vi "AOL Properties parser.vi"(0 "AOL Properties":T4={"AOD 1 thickness (mm)"=118.0, "AOD 2 thickness (mm)"=115.0, "AOD 3 thickness (mm)"=110.0, "AOD 4 thickness (mm)"=135.0, "AOD 5 thickness (mm)"=135.0, "AOD 6 thickness (mm)"=135.0, "AOD 1-2 separation (mm)"=15.0, "AOD 2-3 separation (mm)"=15.0, "AOD 3-4 separation (mm)"=15.0, "AOD 4-5 separation (mm)"=15.0, "AOD 5-6 separation (mm)"=15.0, "AOD 1 X Offset"=15.0, "AOD 2 X Offset"=1.0, "AOD 3 X Offset"=1.0, "AOD 4 X Offset"=1.0, "AOD 1 Y Offset"=1.0, "AOD 2 Y Offset"=1.0, "AOD 3 Y Offset"=1.0, "AOD 4 Y Offset"=1.0, "AOD 1 X Direction"=0.0, "AOD 2 X Direction"=0.0, "AOD 3 X Direction"=0.0, "AOD 4 X Direction"=0.0, "AOD 1 Y Direction"=1.0, "AOD 2 Y Direction"=0.0, "AOD 3 Y Direction"=0.0023, "AOD 4 Y Direction"=0.0046, "AOD 1 Centre (mm)"=15.0, "AOD 2 Centre (mm)"=50.0, "AOD 3 Centre (mm)"=50.0, "AOD 4 Centre (mm)"=50.0, "Timing Offset AOD 1"=0.0, "Timing Offset AOD 2"=0.0, "Timing Offset AOD 3"=0.0, "Timing Offset AOD 4"=0.0, "AOD Optical offset 1"=20000.0, "AOD Optical offset 2"=20000.0, "AOL aperture (mm)"=15.0, "AOL centre wavelength (nm)"=1.0, "AOL centre frequency (MHz)"=1.0, "Diffraction mode"=1.0, "Crystal length (mm)"=0.0, "Acoustic velocity (m/s)"=1.0, "Pair deflection ratio"=1.0, "AOD fill time (us)"=1.0, "AOD Ord. Refractive index"=2.22, "AOD ExtraOrd. Refractive index"=2.22}) -> (14 "Keys setup.DBL":T2=[{"key"="Control FPGA.Clock Freq (MHz)", "Save?"=TRUE, "Default"=240.0}, {"key"="DAQ FPGA.Clock Freq (MHz)", "Save?"=TRUE, "Default"=240.0}], 15 "Values.DBL":dbl[](array[numeric]), 16 "Keys setup.String":T3=[{"key"="Control FPGA.MAC address", "Save?"=TRUE, "Default"="AABBCCDDEEFF"}, {"key"="DAQ FPGA.Target", "Save?"=TRUE, "Default"="RIO0"}, {"key"="XY Stage.COM port", "Save?"=TRUE, "Default"="COM7"}, {"key"="DAQmx Chan.Pockels Control", "Save?"=TRUE, "Default"=""}, {"key"="DAQmx Chan.Hard Shutter", "Save?"=TRUE, "Default"=""}, {"key"="DAQmx Chan.PMT 1", "Save?"=TRUE, "Default"=""}, {"key"="DAQmx Chan.PMT 2", "Save?"=TRUE, "Default"=""}, {"key"="DAQmx Chan.Encoder Trigger", "Save?"=TRUE, "Default"=""}, {"key"="DAQmx Chan.Optional Trigger 1", "Save?"=TRUE, "Default"=""}, {"key"="DAQmx Chan.Optional Trigger 2", "Save?"=TRUE, "Default"=""}, {"key"="DAQmx Chan.Optional Trigger 3", "Save?"=TRUE, "Default"=""}], 17 "Values.Strings":string[](array[string]), 18 "Keys setup.Boolean":T1, 19 "Values.Boolean":bool[](array[boolean]))   [LabVIEW 2017]
uses:
  Typedefs/AOL Properties Cluster.ctl
  Typedefs/Ini file interface (String).ctl
  Typedefs/Ini file interface (DBL).ctl
  Typedefs/Ini file interface (Boolean).ctl
panel:
  # "NOTES:\n1. \"Control FPGA.Ethernet port\" is detected automatically. It is not saved/loaded from file.\n2. \"Control FPGA.Ethernet Opened\" is detected automatically. It is not saved/loaded from file."
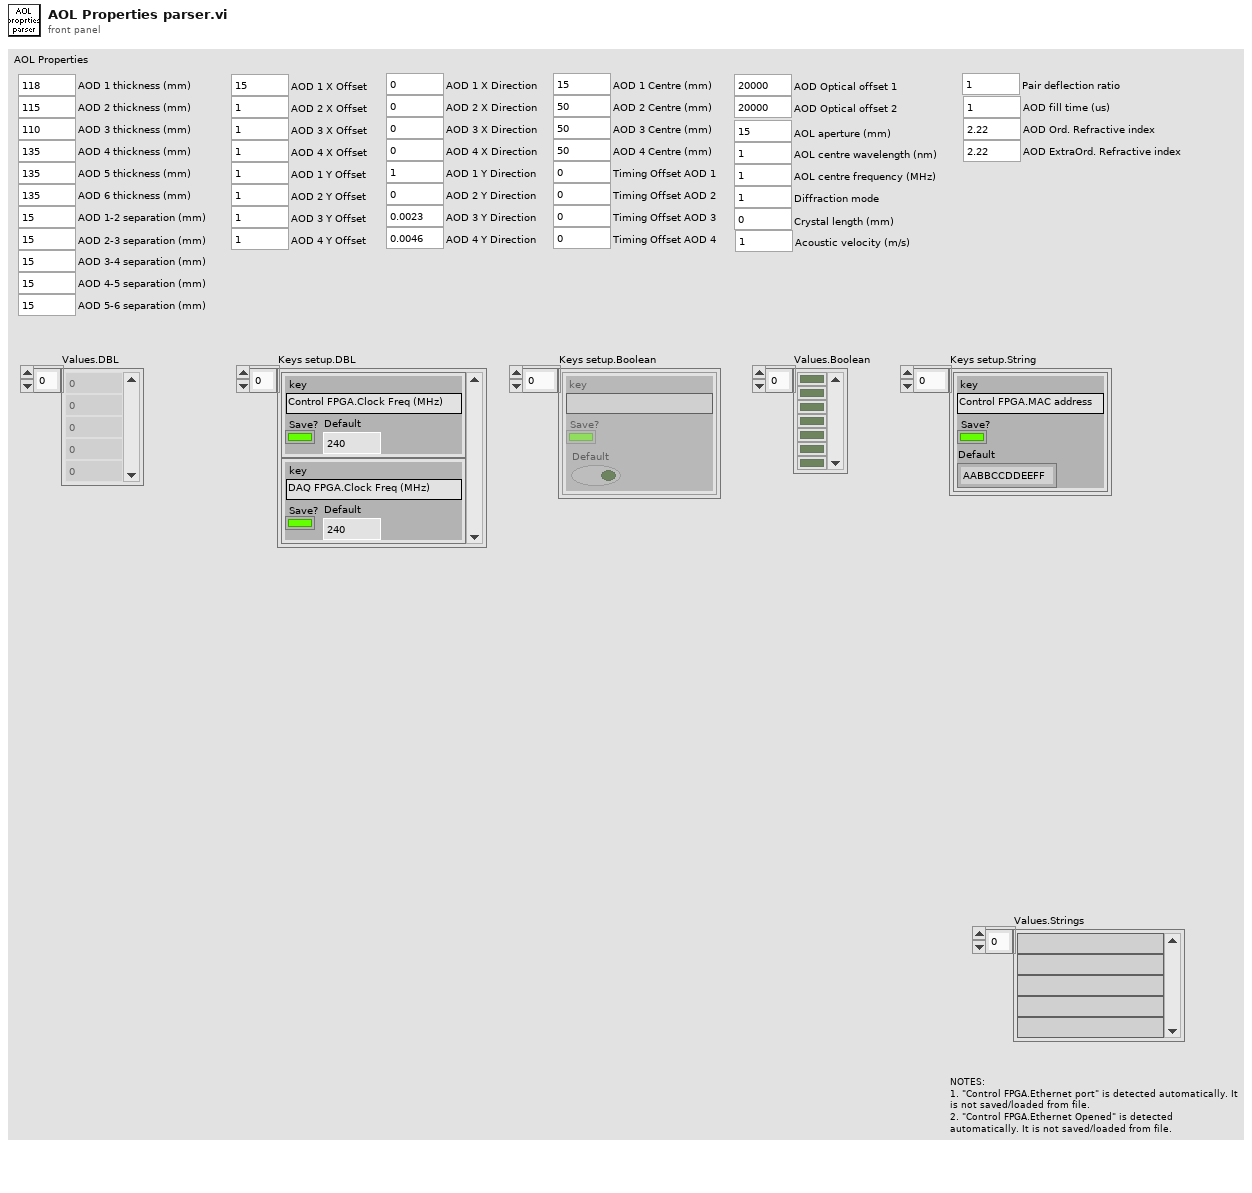
[diagram p1: front panel]
types:
  T1 = typedef "Ini file interface (Boolean).ctl" = cluster{"key":string, "Save?":bool, "Default":bool}[]
  T2 = typedef "Ini file interface (DBL).ctl" = cluster{"key":string, "Save?":bool, "Default":dbl}[]
  T3 = typedef "Ini file interface (String).ctl" = cluster{"key":string, "Save?":bool, "Default":string}[]
  T4 = typedef "AOL Properties Cluster.ctl" = cluster{"AOD 1 thickness (mm)":dbl, "AOD 2 thickness (mm)":dbl, "AOD 3 thickness (mm)":dbl, "AOD 4 thickness (mm)":dbl, "AOD 5 thickness (mm)":dbl, "AOD 6 thickness (mm)":dbl, "AOD 1-2 separation (mm)":dbl, "AOD 2-3 separation (mm)":dbl, "AOD 3-4 separation (mm)":dbl, "AOD 4-5 separation (mm)":dbl, "AOD 5-6 separation (mm)":dbl, "AOD 1 X Offset":dbl, "AOD 2 X Offset":dbl, "AOD 3 X Offset":dbl, "AOD 4 X Offset":dbl, "AOD 1 Y Offset":dbl, "AOD 2 Y Offset":dbl, "AOD 3 Y Offset":dbl, "AOD 4 Y Offset":dbl, "AOD 1 X Direction":dbl, "AOD 2 X Direction":dbl, "AOD 3 X Direction":dbl, "AOD 4 X Direction":dbl, "AOD 1 Y Direction":dbl, "AOD 2 Y Direction":dbl, "AOD 3 Y Direction":dbl, "AOD 4 Y Direction":dbl, "AOD 1 Centre (mm)":dbl, "AOD 2 Centre (mm)":dbl, "AOD 3 Centre (mm)":dbl, "AOD 4 Centre (mm)":dbl, "Timing Offset AOD 1":dbl, "Timing Offset AOD 2":dbl, "Timing Offset AOD 3":dbl, "Timing Offset AOD 4":dbl, "AOD Optical offset 1":dbl, "AOD Optical offset 2":dbl, "AOL aperture (mm)":dbl, "AOL centre wavelength (nm)":dbl, "AOL centre frequency (MHz)":dbl, "Diffraction mode":dbl, "Crystal length (mm)":dbl, "Acoustic velocity (m/s)":dbl, "Pair deflection ratio":dbl, "AOD fill time (us)":dbl, "AOD Ord. Refractive index":dbl, "AOD ExtraOrd. Refractive index":dbl}
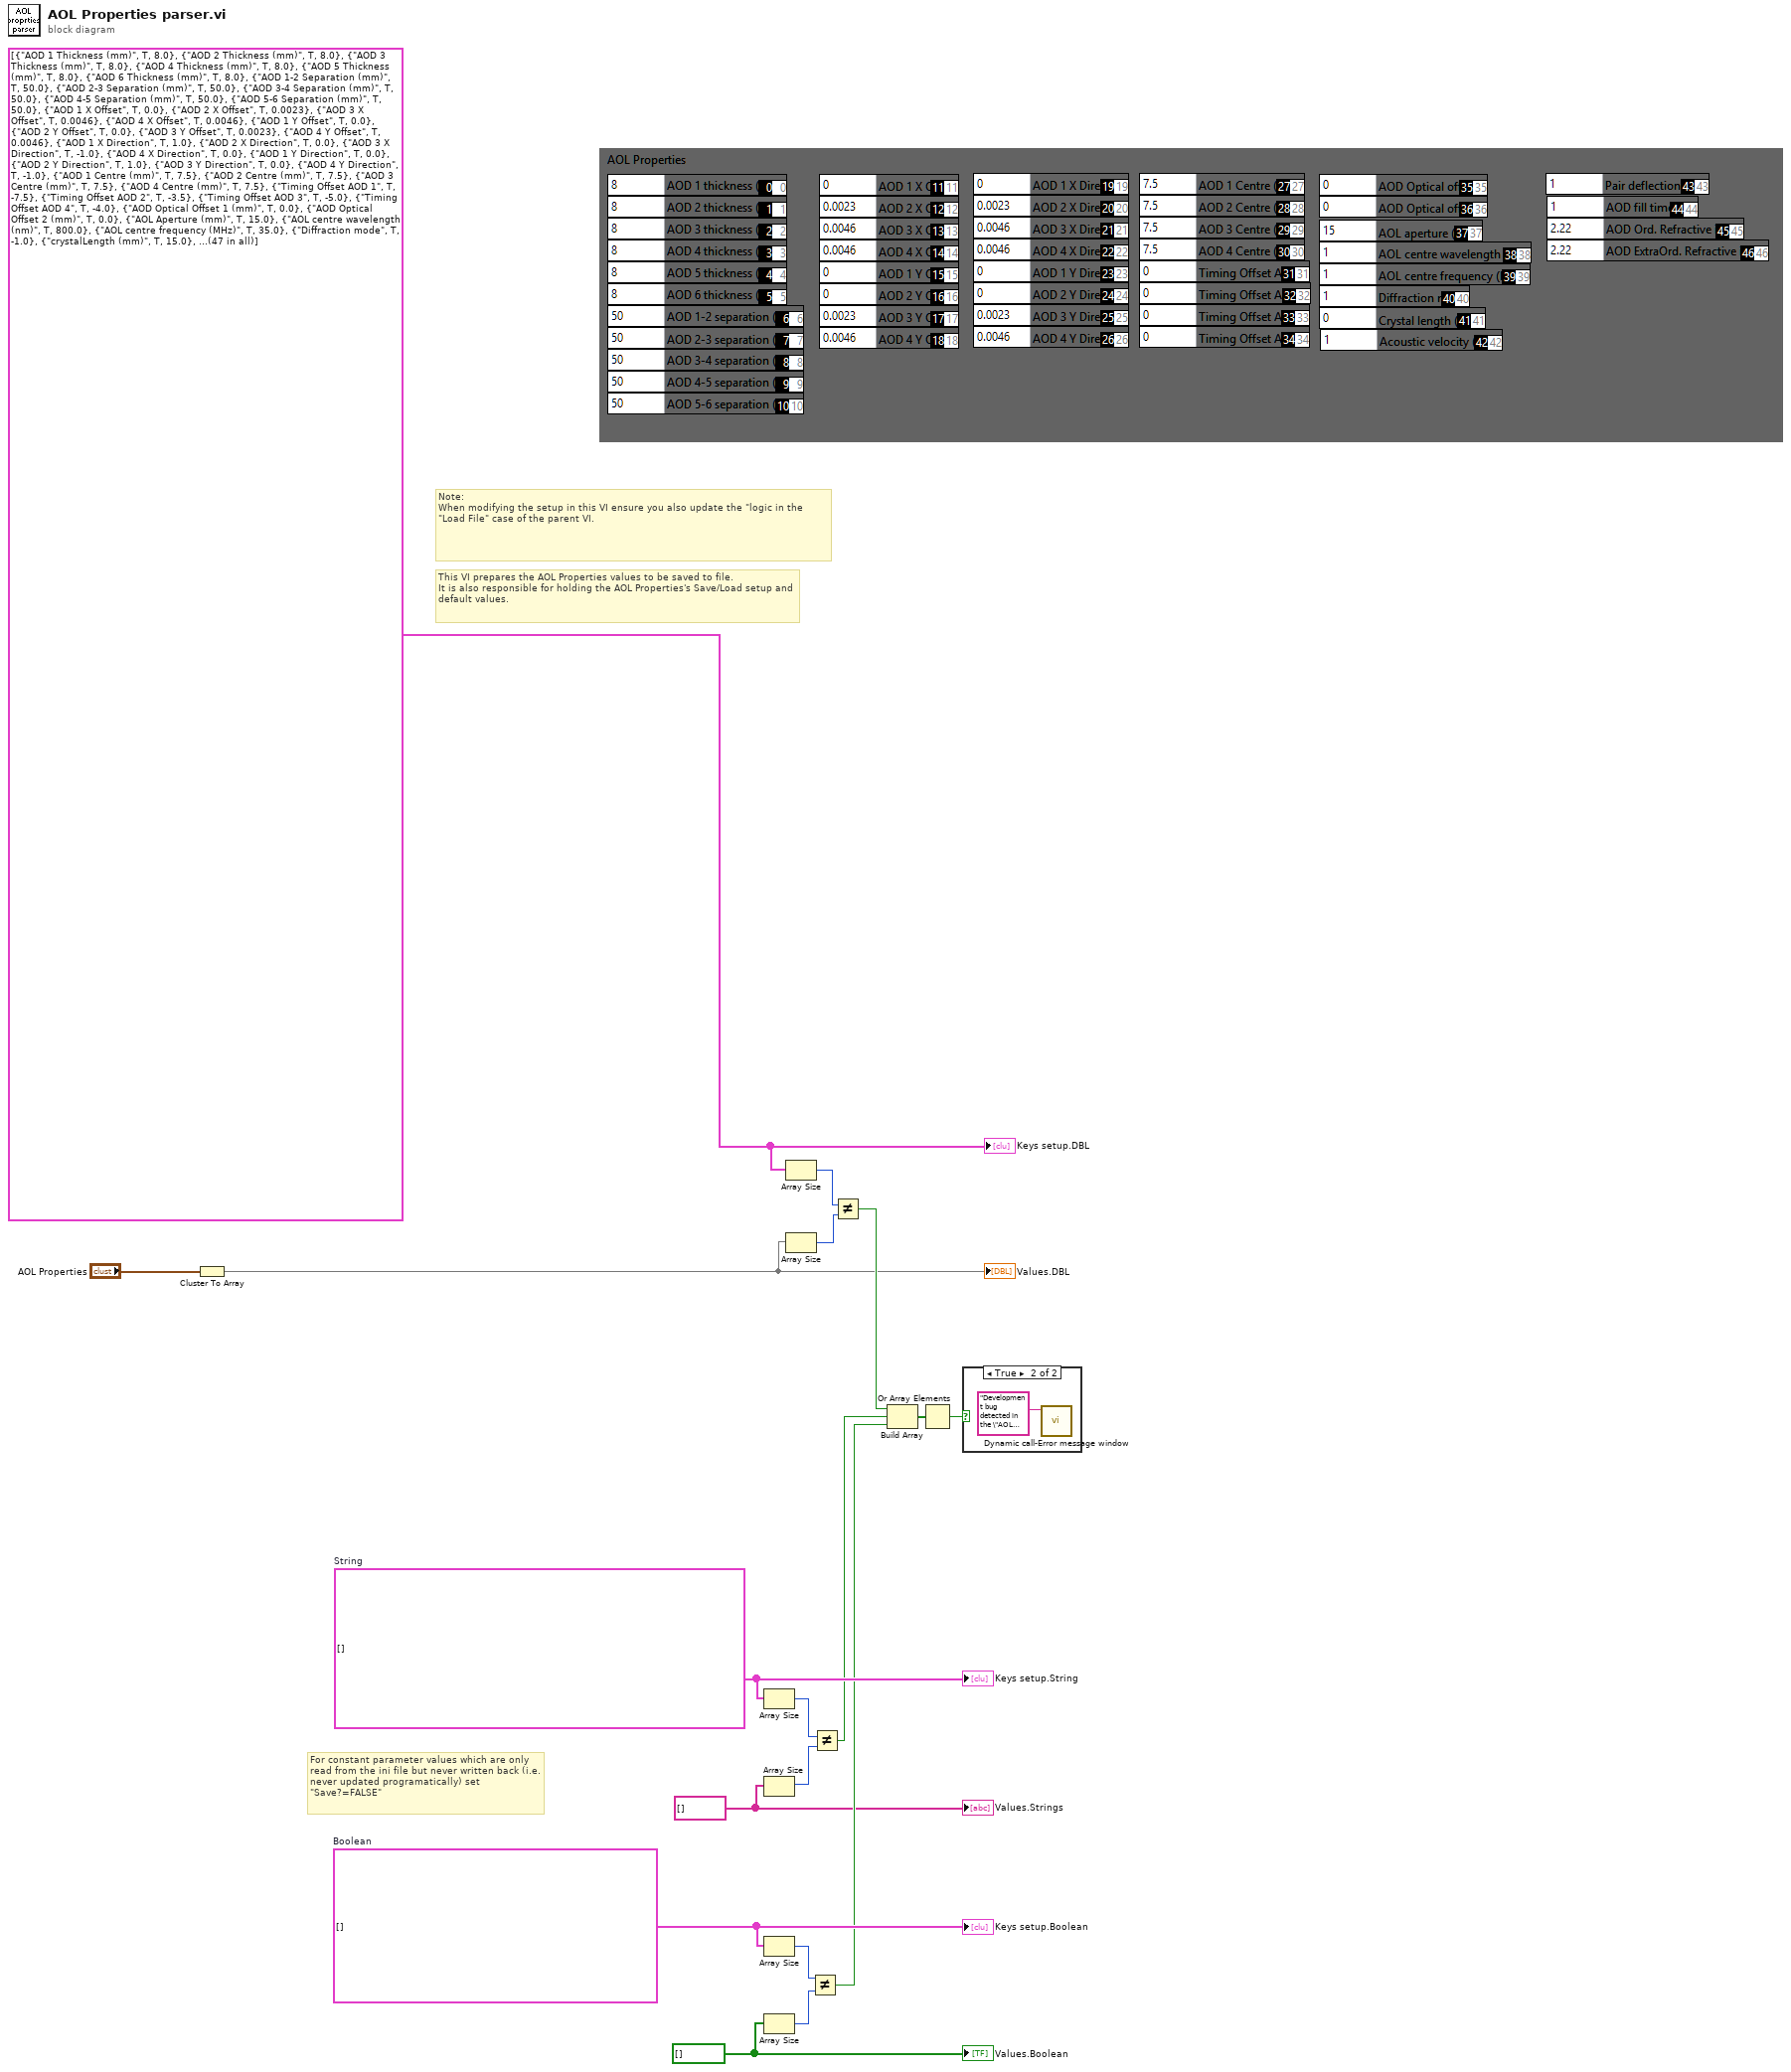
[diagram p0: block diagram]
diagram:
  w3 = T2 [{"key"="AOD 1 Thickness (mm)", "Save?"=TRUE, "Default"=8.0}, {"key"="AOD 2 Thickness (mm)", "Save?"=TRUE, "Default"=8.0}, {"key"="AOD 3 Thickness (mm)", "Save?"=TRUE, "Default"=8.0}, {"key"="AOD 4 Thickness (mm)", "Save?"=TRUE, "Default"=8.0}, {"key"="AOD 5 Thickness (mm)", "Save?"=TRUE, "Default"=8.0}, {"key"="AOD 6 Thickness (mm)", "Save?"=TRUE, "Default"=8.0}, {"key"="AOD 1-2 Separation (mm)", "Save?"=TRUE, "Default"=50.0}, {"key"="AOD 2-3 Separation (mm)", "Save?"=TRUE, "Default"=50.0}, {"key"="AOD 3-4 Separation (mm)", "Save?"=TRUE, "Default"=50.0}, {"key"="AOD 4-5 Separation (mm)", "Save?"=TRUE, "Default"=50.0}, {"key"="AOD 5-6 Separation (mm)", "Save?"=TRUE, "Default"=50.0}, {"key"="AOD 1 X Offset", "Save?"=TRUE, "Default"=0.0}, {"key"="AOD 2 X Offset", "Save?"=TRUE, "Default"=0.0023}, {"key"="AOD 3 X Offset", "Save?"=TRUE, "Default"=0.0046}, {"key"="AOD 4 X Offset", "Save?"=TRUE, "Default"=0.0046}, {"key"="AOD 1 Y Offset", "Save?"=TRUE, "Default"=0.0}, {"key"="AOD 2 Y Offset", "Save?"=TRUE, "Default"=0.0}, {"key"="AOD 3 Y Offset", "Save?"=TRUE, "Default"=0.0023}, {"key"="AOD 4 Y Offset", "Save?"=TRUE, "Default"=0.0046}, {"key"="AOD 1 X Direction", "Save?"=TRUE, "Default"=1.0}, {"key"="AOD 2 X Direction", "Save?"=TRUE, "Default"=0.0}, {"key"="AOD 3 X Direction", "Save?"=TRUE, "Default"=-1.0}, {"key"="AOD 4 X Direction", "Save?"=TRUE, "Default"=0.0}, {"key"="AOD 1 Y Direction", "Save?"=TRUE, "Default"=0.0}, {"key"="AOD 2 Y Direction", "Save?"=TRUE, "Default"=1.0}, {"key"="AOD 3 Y Direction", "Save?"=TRUE, "Default"=0.0}, {"key"="AOD 4 Y Direction", "Save?"=TRUE, "Default"=-1.0}, {"key"="AOD 1 Centre (mm)", "Save?"=TRUE, "Default"=7.5}, {"key"="AOD 2 Centre (mm)", "Save?"=TRUE, "Default"=7.5}, {"key"="AOD 3 Centre (mm)", "Save?"=TRUE, "Default"=7.5}, {"key"="AOD 4 Centre (mm)", "Save?"=TRUE, "Default"=7.5}, {"key"="Timing Offset AOD 1", "Save?"=TRUE, "Default"=-7.5}, {"key"="Timing Offset AOD 2", "Save?"=TRUE, "Default"=-3.5}, {"key"="Timing Offset AOD 3", "Save?"=TRUE, "Default"=-5.0}, {"key"="Timing Offset AOD 4", "Save?"=TRUE, "Default"=-4.0}, {"key"="AOD Optical Offset 1 (mm)", "Save?"=TRUE, "Default"=0.0}, {"key"="AOD Optical Offset 2 (mm)", "Save?"=TRUE, "Default"=0.0}, {"key"="AOL Aperture (mm)", "Save?"=TRUE, "Default"=15.0}, {"key"="AOL centre wavelength (nm)", "Save?"=TRUE, "Default"=800.0}, {"key"="AOL centre frequency (MHz)", "Save?"=TRUE, "Default"=35.0}, {"key"="Diffraction mode", "Save?"=TRUE, "Default"=-1.0}, {"key"="crystalLength (mm)", "Save?"=TRUE, "Default"=15.0}, {"key"="Acoustic velocity (m/s)", "Save?"=TRUE, "Default"=613.0}, {"key"="Pair Deflection Ratio", "Save?"=TRUE, "Default"=1.0}, {"key"="AOD fill time (us)", "Save?"=TRUE, "Default"=24.5}, {"key"="AOD Ord. Refractive index", "Save?"=TRUE, "Default"=2.22}, {"key"="AOD ExtraOrd. Refractive index", "Save?"=TRUE, "Default"=2.44}] ("DBL 3")
  w4 = bool[] [] ("appended array")
  w5 = string[] [] ("appended array")
  w17 = T1 []  # Boolean
  w18 = T3 []  # String
  # "Note:\nWhen modifying the setup in this VI ensure you also update the \"logic in the \"Load File\" case of the parent VI."
  # "For constant parameter values which are only read from the ini file but never written back (i.e. never updated programatically) set \"Save?=FALSE\""
  # "This VI prepares the AOL Properties values to be saved to file.\nIt is also responsible for holding the AOL Properties's Save/Load setup and default values."
  n1 = Cluster To Array(cluster="AOL Properties") -> (array=w1:dbl[])
  "Values.DBL" <- w1
  n2 = Array Size(array=w18) -> (size(s)=w16:i32)
  n3 = Array Size(array=w5) -> (size(s)=w15:i32)
  n4 = Array Size(array=w17) -> (size(s)=w12:i32)
  n5 = Array Size(array=w4) -> (size(s)=w11:i32)
  n6 = Array Size(array=w3) -> (size(s)=w14:i32)
  n7 = Array Size(array=w1) -> (size(s)=w13:i32)
  n8 = Not Equal?(x=w12, y=w11) -> (x != y?=w9:bool)
  n9 = Not Equal?(x=w16, y=w15) -> (x != y?=w6:bool)
  n10 = Not Equal?(x=w14, y=w13) -> (x != y?=w7:bool)
  n11 = Build Array(w7, w6, w9) -> (w10:bool[])
  n12 = Or Array Elements(Boolean array=w10) -> (logical OR=w8:bool)
  n13 = case shown="True" w8 {
    frame False {
    }
    frame True {
      n14 = call "Dynamic call-Error message window.vi"("Error Message"="Development bug detected in the \"AOL properties parser.vi\".\nPlease correct the set up in this VI.") -> ()  [unwired: 10 in, 1 out]
    }
  }
  "Keys setup.String" <- w18
  "Keys setup.DBL" <- w3
  "Values.Strings" <- w5
  "Keys setup.Boolean" <- w17
  "Values.Boolean" <- w4
